vi "Solve1.vi"(8 "Error In":errorcluster, 11 "object in":refnum<class "2021_25.lvclass">) -> (0 "Error Out":errorcluster, 2 "Result":u64, 3 "object out":refnum<class "2021_25.lvclass">)   [LabVIEW 2020, in "2021_25.lvclass"]
uses:
  2021_25.lvclass
  2021_25.lvclass/2021_25.ctl
panel:
  out "Start":string[][](array[string])
  out "Before":string[][](array[string])
  out "After":string[][](array[string])
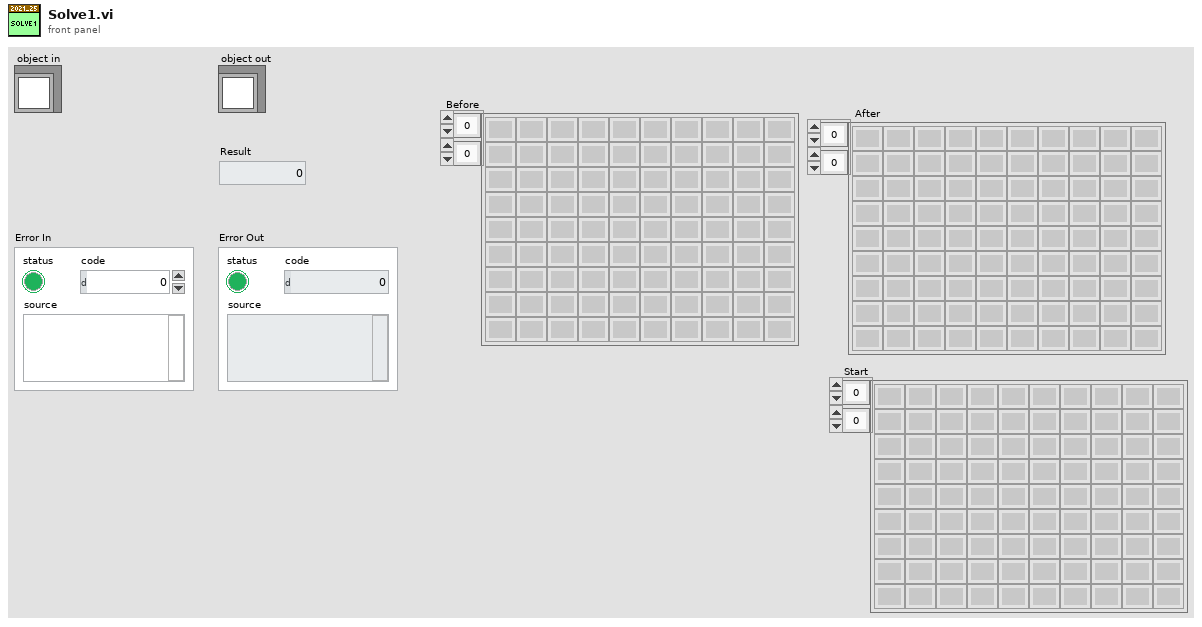
[diagram p1: front panel]
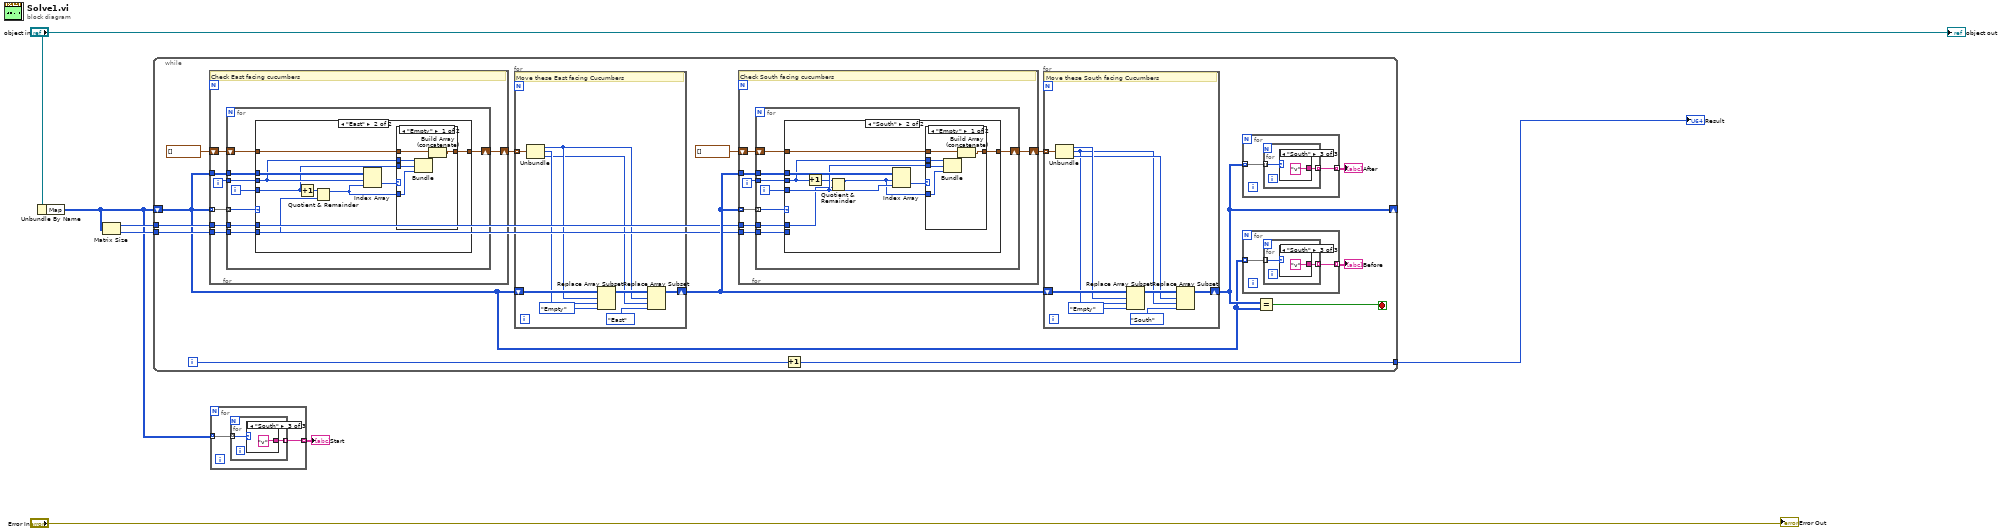
[diagram p0: block diagram]
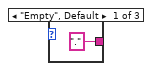
[diagram p2: hidden frame]
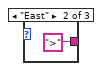
[diagram p3: hidden frame]
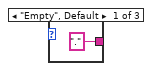
[diagram p6: hidden frame]
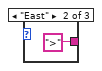
[diagram p7: hidden frame]
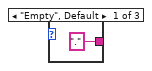
[diagram p8: hidden frame]
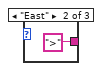
[diagram p9: hidden frame]
diagram:
  n1 = Unbundle By Name("object in") -> ("Map"=w1:enum16{"Empty", "East", "South"}[][])
  n2 = Matrix Size(0:w1) -> (1:w5:i32, 2:w4:i32)
  n3 = while {
    tunnel: w5 -> [w12]
    tunnel: w4 -> [w11]
    tunnel: [w8] -> w3
    shift-right: [w10] -> _
    shift-left: w1 -> [w9]
    i -> [w20]
    stop <- w21 stop-if-true
    n4 = for {
      tunnel: w9 -> [w92] mode=indexing
      tunnel: w9 -> [w91]
      tunnel: w12 -> [w89]
      tunnel: w11 -> [w88]
      shift-right: [w86] -> w17
      shift-left: cluster{"Row":i32, "Column":i32, "Next":i32}[] [] -> [w87]
      i -> [w90]
      # "Check East facing cucumbers"
      n5 = for {
        tunnel: w92 -> [w100] mode=indexing
        tunnel: w91 -> [w99]
        tunnel: w90 -> [w98]
        tunnel: w89 -> [w96]
        tunnel: w88 -> [w95]
        shift-right: [w93] -> w86
        shift-left: w87 -> [w94]
        i -> [w97]
        n6 = case shown="\"East\"" w100 {
          tunnel: w99 -> [_ w110]
          tunnel: w98 -> [_ w105]
          tunnel: w97 -> [_ w104]
          tunnel: w96 -> [_ _]
          tunnel: w95 -> [_ w109]
          tunnel: w94 -> [w101 w107]
          tunnel: [w101 w106] -> w93
          frame Default {
          }
          frame "East" {
            n7 = Increment(x=w104) -> (x+1=w103:i32)
            n8 = Quotient & Remainder(x=w103, y=w109) -> (x-y*floor(x/y)=w102:i32)  [unwired: 1 out]
            n9 = Index Array(array=w110, index (row)=w105, index (col)=w102) -> (element=w108:enum16{"Empty", "East", "South"})
            n10 = case shown="\"Empty\"" w108 {
              tunnel: w107 -> [w116 w117]
              tunnel: [w115 w117] -> w106
              tunnel: w105 -> [w114 _]
              tunnel: w102 -> [w113 _]
              tunnel: w104 -> [w111 _]
              frame "Empty" {
                n11 = Bundle(w114, w111, w113) -> (w112:cluster{i32, i32, i32})  [unwired: 1 in]
                n12 = Build Array (concatenate)(w116, w112) -> (w115:cluster{"Row":i32, "Column":i32, "Next":i32}[])
              }
              frame Default {
              }
            }
          }
        }
      }
    }
    n13 = for {
      shift-right: [w65] -> w13
      shift-left: w9 -> [w71]
      tunnel: w17 -> [w70] mode=indexing
      # "Move these East facing Cucumbers"
      n14 = Unbundle(w70) -> ("Row"=w64:i32, "Column"=w67:i32, "Next"=w63:i32)
      n15 = Replace Array Subset(array=w71, new element=enum16{"Empty", "East", "South"}."Empty" ("new element/subarray"), index (row)=w64, index (col)=w67) -> (w68:enum16{"Empty", "East", "South"}[][])
      n16 = Replace Array Subset(array=w68, new element=enum16{"Empty", "East", "South"}."East" ("new element/subarray"), index (row)=w64, index (col)=w63) -> (w65:enum16{"Empty", "East", "South"}[][])
    }
    n17 = for {
      tunnel: w13 -> [w37] mode=indexing
      tunnel: w13 -> [w36]
      tunnel: w12 -> [w34]
      tunnel: w11 -> [w33]
      shift-right: [w31] -> w14
      shift-left: cluster{"Row":i32, "Column":i32, "Next":i32}[] [] -> [w32]
      i -> [w35]
      # "Check South facing cucumbers"
      n18 = for {
        tunnel: w37 -> [w45] mode=indexing
        tunnel: w36 -> [w44]
        tunnel: w35 -> [w43]
        tunnel: w34 -> [w41]
        tunnel: w33 -> [w40]
        shift-right: [w38] -> w31
        shift-left: w32 -> [w39]
        i -> [w42]
        n19 = case shown="\"South\"" w45 {
          tunnel: w44 -> [_ w55]
          tunnel: w43 -> [_ w50]
          tunnel: w42 -> [_ w51]
          tunnel: w41 -> [_ w49]
          tunnel: w40 -> [_ _]
          tunnel: w39 -> [w46 w53]
          tunnel: [w46 w52] -> w38
          frame Default {
          }
          frame "South" {
            n20 = Increment(x=w50) -> (x+1=w48:i32)
            n21 = Quotient & Remainder(x=w48, y=w49) -> (x-y*floor(x/y)=w47:i32)  [unwired: 1 out]
            n22 = Index Array(array=w55, index (row)=w47, index (col)=w51) -> (element=w54:enum16{"Empty", "East", "South"})
            n23 = case shown="\"Empty\"" w54 {
              tunnel: w53 -> [w61 w62]
              tunnel: [w60 w62] -> w52
              tunnel: w50 -> [w59 _]
              tunnel: w47 -> [w58 _]
              tunnel: w51 -> [w56 _]
              frame "Empty" {
                n24 = Bundle(w59, w56, w58) -> (w57:cluster{i32, i32, i32})  [unwired: 1 in]
                n25 = Build Array (concatenate)(w61, w57) -> (w60:cluster{"Row":i32, "Column":i32, "Next":i32}[])
              }
              frame Default {
              }
            }
          }
        }
      }
    }
    n26 = Increment(x=w20) -> (x+1=w8:i32)
    n27 = for {
      shift-right: [w22] -> w10
      shift-left: w13 -> [w30]
      tunnel: w14 -> [w29] mode=indexing
      # "Move these South facing Cucumbers"
      n28 = Unbundle(w29) -> ("Row"=w28:i32, "Column"=w24:i32, "Next"=w25:i32)
      n29 = Replace Array Subset(array=w30, new element=enum16{"Empty", "East", "South"}."Empty" ("new element/subarray"), index (row)=w28, index (col)=w24) -> (w26:enum16{"Empty", "East", "South"}[][])
      n30 = Replace Array Subset(array=w26, new element=enum16{"Empty", "East", "South"}."South" ("new element/subarray"), index (row)=w25, index (col)=w24) -> (w22:enum16{"Empty", "East", "South"}[][])
    }
    n31 = for {
      tunnel: [w80] -> w19 mode=indexing
      tunnel: w10 -> [w79] mode=indexing
      n32 = for {
        tunnel: [w82] -> w80 mode=indexing
        tunnel: w79 -> [w81] mode=indexing
        n33 = case shown="\"South\"" w81 {
          tunnel: ["." ">" "v"] -> w82
          frame "Empty", Default {
          }
          frame "East" {
          }
          frame "South" {
          }
        }
      }
    }
    "After" <- w19
    n34 = for {
      tunnel: [w73] -> w18 mode=indexing
      tunnel: w9 -> [w72] mode=indexing
      n35 = for {
        tunnel: [w75] -> w73 mode=indexing
        tunnel: w72 -> [w74] mode=indexing
        n36 = case shown="\"South\"" w74 {
          tunnel: ["." ">" "v"] -> w75
          frame "Empty", Default {
          }
          frame "East" {
          }
          frame "South" {
          }
        }
      }
    }
    "Before" <- w18
    n37 = Equal?(x=w10, y=w9) -> (x = y?=w21:bool)
  }
  "Result" <- w3
  n38 = for {
    tunnel: w1 -> [w119] mode=indexing
    tunnel: [w118] -> w2 mode=indexing
    n39 = for {
      tunnel: w119 -> [w121] mode=indexing
      tunnel: [w120] -> w118 mode=indexing
      n40 = case shown="\"South\"" w121 {
        tunnel: ["." ">" "v"] -> w120
        frame "Empty", Default {
        }
        frame "East" {
        }
        frame "South" {
        }
      }
    }
  }
  "Start" <- w2
  "Error Out" <- "Error In"
  "object out" <- "object in"
